vi "Configure Hardware - Copie.vi"(8 "error in (no error)":errorcluster, 11 "Hardware Resources in":T1) -> (0 "error out":errorcluster, 3 "Hardware Resources out":T1)   [LabVIEW 2018, in "Acquisition.lvlib"]
doc: "Configure the hardware."
uses:
  Acquisition.lvlib
  Hardware Configuration.ctl
  <vilib>/DAQmx/create/channels.llb/DAQmx Create Channel (AI-Voltage-Basic).vi
  <vilib>/DAQmx/configure/timing.llb/DAQmx Timing (Sample Clock).vi
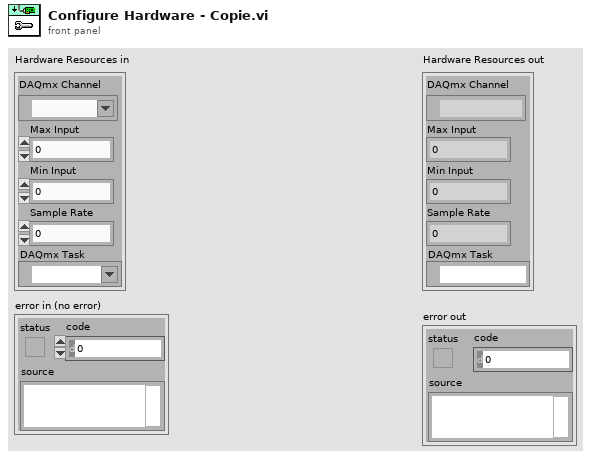
[diagram p1: front panel]
types:
  T1 = typedef "Acquisition.lvlib/Hardware Configuration.ctl" = cluster{"DAQmx Channel":tag, "Max Input":dbl, "Min Input":dbl, "Sample Rate":dbl, "DAQmx Task":refnum<k21>}
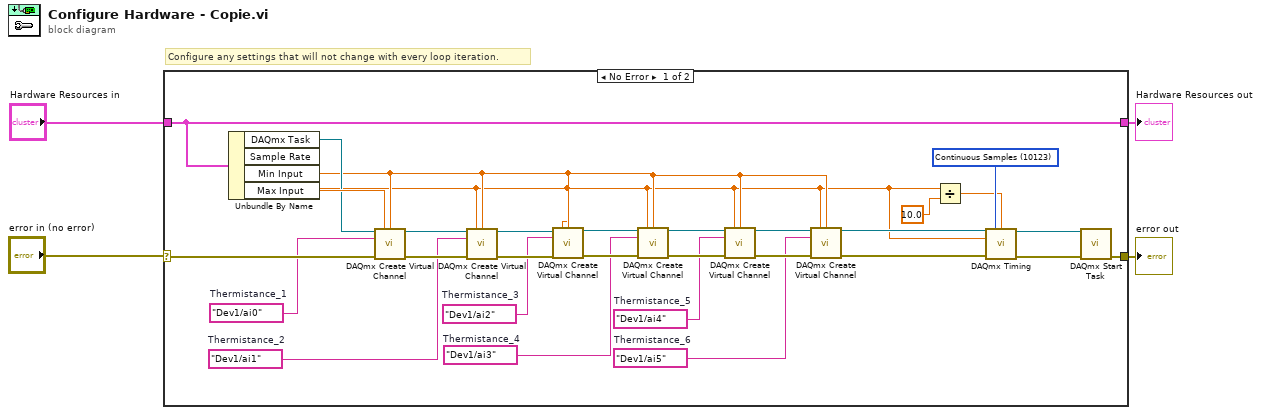
[diagram p0: block diagram]
diagram:
  # "Configure any settings that will not change with every loop iteration."
  n1 = case shown="No Error" "error in (no error)" {
    selector: "error in (no error)" -> [w33 w35]
    tunnel: [w26 w35] -> w3
    tunnel: "Hardware Resources in" -> [w32 w36]
    tunnel: [w32 w36] -> w1
    frame No Error {
      w5 = tag "Dev1/ai5"  # Thermistance_6
      w6 = tag "Dev1/ai4"  # Thermistance_5
      w7 = tag "Dev1/ai3"  # Thermistance_4
      w8 = tag "Dev1/ai2"  # Thermistance_3
      w9 = tag "Dev1/ai1"  # Thermistance_2
      w10 = tag "Dev1/ai0"  # Thermistance_1
      w31 = 10123 items=["Finite Samples"=10178, "Continuous Samples"=10123, "Hardware Timed Single Point"=12522] ("sample mode")
      n2 = Unbundle By Name(w32) -> ("DAQmx Task"=w25:refnum<k21>, "Sample Rate"=w11:dbl, "Min Input"=w12:dbl, "Max Input"=w34:dbl)
      n3 = call-poly <vilib>:"DAQmx Create Virtual Channel.vi"("task in"=w25, "maximum value"=w34, "minimum value"=w12, "physical channels"=w10, "error in"=w33) -> ("task out"=w24:refnum<k21>, "error out"=w23:errorcluster)  [unwired: 9 in]
      n4 = call-poly <vilib>:"DAQmx Create Virtual Channel.vi"("task in"=w24, "maximum value"=w11, "minimum value"=w12, "physical channels"=w9, "error in"=w23) -> ("task out"=w22:refnum<k21>, "error out"=w21:errorcluster)  [unwired: 9 in]
      n5 = call-poly <vilib>:"DAQmx Create Virtual Channel.vi"("task in"=w22, "maximum value"=w11, "minimum value"=w12, "physical channels"=w8, "error in"=w21) -> ("task out"=w20:refnum<k21>, "error out"=w19:errorcluster)  [unwired: 9 in]
      n6 = call-poly <vilib>:"DAQmx Create Virtual Channel.vi"("task in"=w20, "maximum value"=w11, "minimum value"=w12, "physical channels"=w7, "error in"=w19) -> ("task out"=w18:refnum<k21>, "error out"=w17:errorcluster)  [unwired: 9 in]
      n7 = call-poly <vilib>:"DAQmx Create Virtual Channel.vi"("task in"=w18, "maximum value"=w11, "minimum value"=w12, "physical channels"=w6, "error in"=w17) -> ("task out"=w16:refnum<k21>, "error out"=w14:errorcluster)  [unwired: 9 in]
      n8 = call-poly <vilib>:"DAQmx Create Virtual Channel.vi"("task in"=w16, "maximum value"=w11, "minimum value"=w12, "physical channels"=w5, "error in"=w14) -> ("task out"=w15:refnum<k21>, "error out"=w13:errorcluster)  [unwired: 9 in]
      n9 = Divide(x=w11, y=10.0) -> (x/y=w29:dbl)
      n10 = call-poly <vilib>:"DAQmx Timing.vi"("task/channels in"=w15, "sample mode"=w31, "samples per channel"=w29, "rate"=w11, "error in"=w13) -> ("task out"=w27:refnum<k21>, "error out"=w28:errorcluster)  [unwired: 9 in]
      n11 = call <vilib>:"DAQmx Start Task.vi"("task/channels in"=w27, "error in"=w28) -> ("error out"=w26:errorcluster)  [unwired: 12 in, 1 out]
    }
    frame Error {
    }
  }
  "Hardware Resources out" <- w1
  "error out" <- w3
